vi "currentPeak.vi"(8 "error in (no error)":errorcluster, 10 "Istring# change":string, 11 "Istring# scan":string) -> (0 "error out":errorcluster, 2 "Ipeak":string, 3 "Irun":string)   [LabVIEW 2018]
uses:
  Global_usbComm.vi
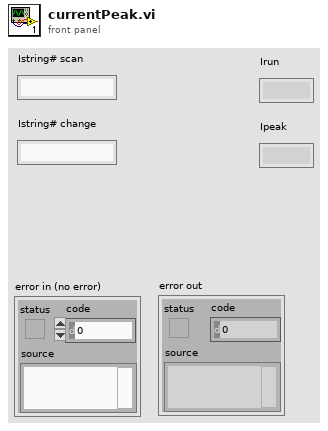
[diagram p1: front panel]
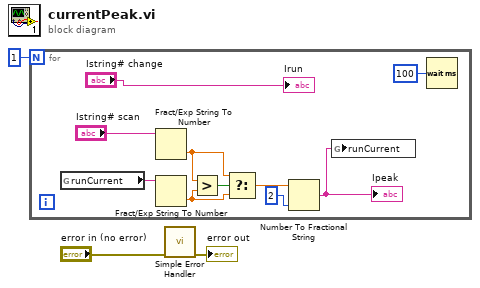
[diagram p0: block diagram]
diagram:
  n1 = for {
    N: 1 -> [_]
    n2 = global read "Global_usbComm.vi" "runCurrent"() -> (w12:string)
    n3 = Fract/Exp String To Number(string="Istring# scan") -> (number=w7:dbl)  [unwired: 3 in, 1 out]
    n4 = Fract/Exp String To Number(string=w12) -> (number=w11:dbl)  [unwired: 3 in, 1 out]
    n5 = Greater?(x=w7, y=w11) -> (0:w13:bool)
    n6 = Select(t=w7, s=w13, f=w11) -> (s? t:f=w10:dbl)
    n7 = Number To Fractional String(number=w10, precision (6)=i16 2) -> (F-format string=w9:string)  [unwired: 2 in]
    "Ipeak" <- w9
    n8 = global write "Global_usbComm.vi" "runCurrent"(w9) -> ()
    n9 = Wait (ms)(milliseconds to wait=u32 100) -> ()  [unwired: 1 out]
    "Irun" <- "Istring# change"
  }
  n10 = call <vilib>:"Simple Error Handler.vi"("error in (no error)"="error in (no error)") -> ("error out"=→"error out":errorcluster)  [unwired: 4 in, 4 out]
